vi "DAQ Para.vi"() -> (1 "Thread Para":T4={"error"={"status"=FALSE, "code"=0, "source"=""}, "LocalQ"={"LQName"="", "LQEvent"="", "LQData"=variant}, "HighQ"={"HQName"="", "HQEvent"="", "HQData"=variant}, "Channel"={"CHTag*"="", "Used?*"=FALSE, "CHName"="", "Unit"="MPa", "斜率"=0.0, "截距"=0.0}, "Card"={"Module Type"="", "Module Name"="", "ModuSN"="", "ModuIP"="", "Used?"=FALSE, "Connected"=FALSE, "Timing*"={"Sample Rate"=1000.0}, "Channels"=[]}, "hwType"="", "hwDriverRef"={"DevicesAndSignals"={"Devices"=[], "Signals"=[]}, "DaqMeasurement"=refnum}, "DevsInfo"=[], "DataQ"="", "tdms ref"=refnum, "Save"=FALSE, "T0"=timestamp(0 s since 1904-01-01)})   [LabVIEW 2016]
uses:
  DAQ-Config/Controls/PSCHN_Channel Para.ctl
  DAQ-Config/Controls/PSCHN_Card Para.ctl
  Hardware Drivers/QX/hw_QX_hwDriverRef.ctl
  C:/Users/CL/Desktop/ZcDAQprj0811/ZcDAQprj/Modules/DAQ-Device/Hardware Drivers/QX/HBM LabVIEW Driver/DLLs/Hbm.Api.Common.dll
  Hardware Drivers/QX/HBM LabVIEW Driver/DLLs/Hbm.Api.Common.dll
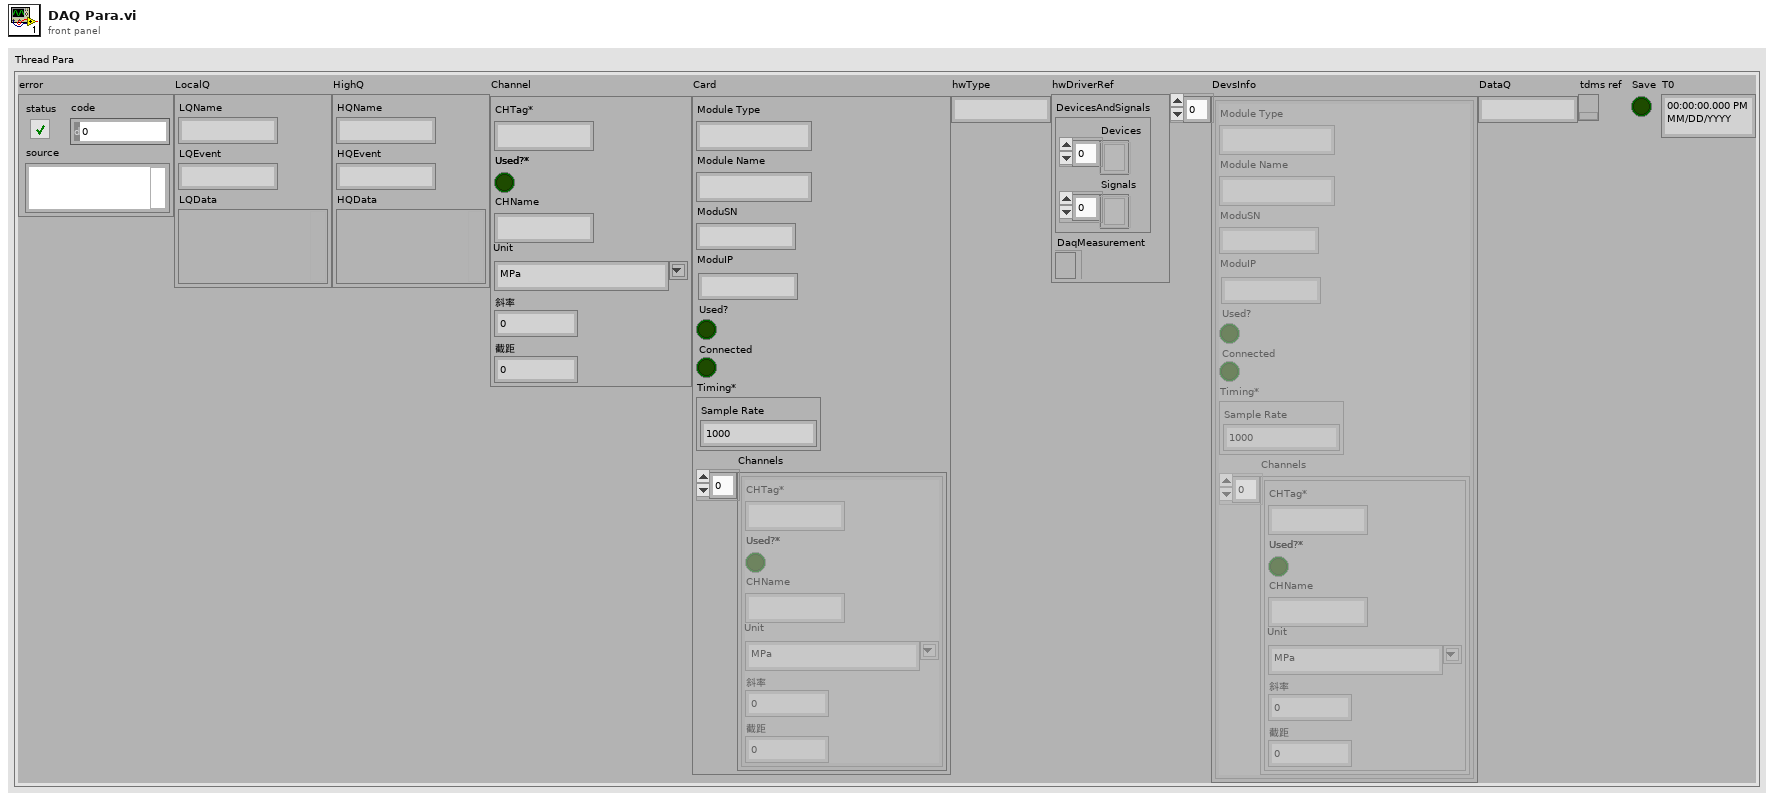
[diagram p1: front panel]
types:
  T1 = typedef "PSCHN_Channel Para.ctl" = cluster{"CHTag*":string, "Used?*":bool, "CHName":string, "Unit":string, "斜率":dbl, "截距":dbl}
  T2 = typedef "PSCHN_Card Para.ctl" = cluster{"Module Type":string, "Module Name":string, "ModuSN":string, "ModuIP":string, "Used?":bool, "Connected":bool, "Timing*":cluster{"Sample Rate":dbl}, "Channels":T1[]}
  T3 = typedef "hw_QX_hwDriverRef.ctl" = cluster{"DevicesAndSignals":cluster{"Devices":refnum<k24>[], "Signals":refnum<k24>[]}, "DaqMeasurement":refnum<k24>}
  T4 = cluster{"error":errorcluster, "LocalQ":cluster{"LQName":string, "LQEvent":string, "LQData":variant}, "HighQ":cluster{"HQName":string, "HQEvent":string, "HQData":variant}, "Channel":T1, "Card":T2, "hwType":string, "hwDriverRef":T3, "DevsInfo":T2[], "DataQ":string, "tdms ref":refnum<k34>, "Save":bool, "T0":timestamp}
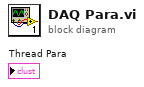
[diagram p0: block diagram]
diagram:
